vi "SDCP Transfer Mode Command.vi"(4 "error in (no error)":errorcluster, 5 "FTOR":bool, 6 "BTR":bool, 7 "SFT":bool) -> (0 "error out":errorcluster)   [LabVIEW 2020]
uses:
  Typedefs/SDCP - Serial Port Control - Commands.ctl
  <vilib>/Instr/_visa.llb/VISA Flush IO Buffer Mask.ctl
panel:
  out "Number of tries":i32
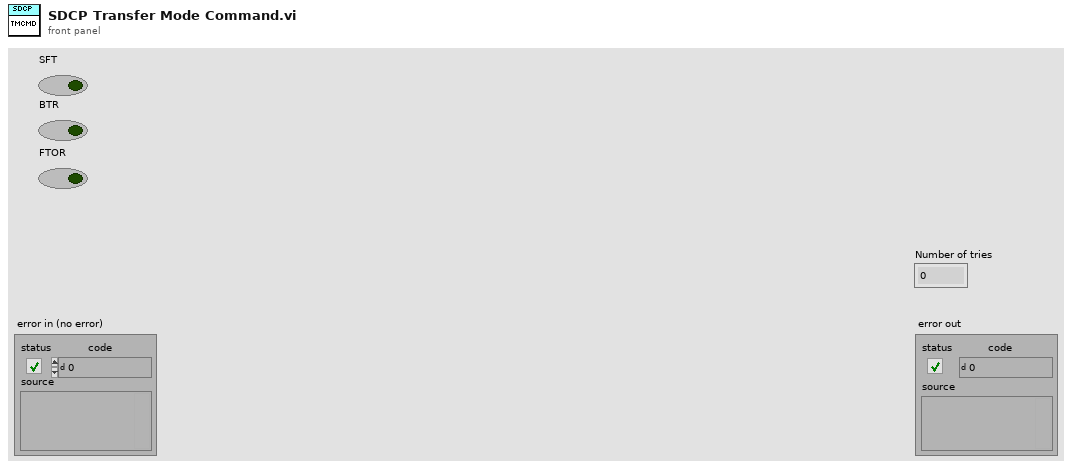
[diagram p1: front panel]
types:
  T1 = typedef "VISA Flush IO Buffer Mask.ctl" = u16
  T2 = typedef "SDCP - Serial Port Control - Commands.ctl" = enum16{"Open", "Read", "Write", "Get instance", "Close"}
  T3 = typedef "SDCP TMC Param.ctl" = cluster{"TMS_REQ":bool, "TMS_ACK":bool, "TMC_REQ":bool, "TMC_ACK":bool, "BTR_ENSTAT":bool, "FTOR_ENSTAT":bool, "SFT_ENSTAT":bool, "BTR_ENREQ":bool, "FTOR_ENREQ":bool, "SFT_ENREQ":bool, "MTR_ENREQ":bool, "MTR_ENACK":bool}
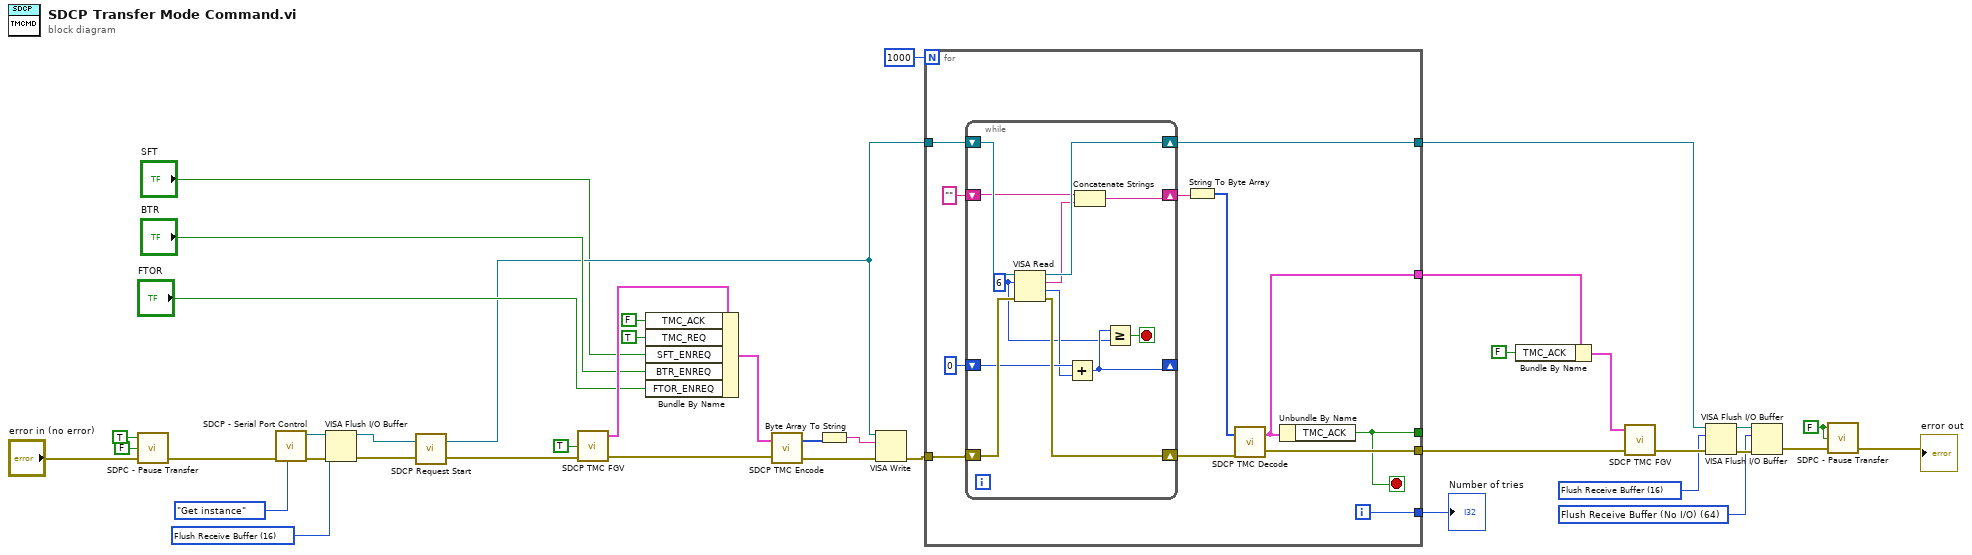
[diagram p0: block diagram]
diagram:
  w2 = FALSE ("Pause transfer")
  w13 = T1 64 items=["Flush Receive Buffer"=16, "Write Transmit Buffer to Device"=32, "Flush Receive Buffer (No I/O)"=64, "Flush Transmit Buffer"=128] ("Mask")
  w16 = T1 16 items=["Flush Receive Buffer"=16, "Write Transmit Buffer to Device"=32, "Flush Receive Buffer (No I/O)"=64, "Flush Transmit Buffer"=128] ("Mask")
  w19 = T1 16 items=["Flush Receive Buffer"=16, "Write Transmit Buffer to Device"=32, "Flush Receive Buffer (No I/O)"=64, "Flush Transmit Buffer"=128] ("Mask")
  n1 = call "SDPC - Pause Transfer.vi"("error in (no error)"="error in (no error)", "RD/nWR"=FALSE, "Pause transfer"=TRUE) -> ("error out"=w10:errorcluster)  [unwired: 1 in, 1 out]
  n2 = call "SDCP - Serial Port Control.vi"("Command"=SDCP_-_Serial_Port_Control_-_Commands."Get instance", "error in (no error)"=w10) -> ("error out"=w21:errorcluster, "VISA out"=w20:refnum<visa-resource-name>)  [unwired: 6 in, 2 out]
  n3 = VISA Flush I/O Buffer(VISA resource name=w20, mask (16)=w19, error in (no error)=w21) -> (VISA resource name out=w6:refnum<visa-resource-name>, error out=w7:errorcluster)
  n4 = call "SDCP Request Start.vi"("error in (no error)"=w7, "COM Port"=w6) -> ("error out"=w4:errorcluster, "COM Port Out"=w5:refnum<visa-resource-name>)
  n5 = call "SDCP TMC FGV.vi"("error in (no error)"=w4, "RD/nWR"=TRUE) -> ("error out"=w33:errorcluster, "TMC out"=w38:T3)  [unwired: 2 in]
  n6 = Bundle By Name(cluster=w38, "TMC_ACK"=FALSE, "TMC_REQ"=TRUE, "SFT_ENREQ"="SFT", "BTR_ENREQ"="BTR", "FTOR_ENREQ"="FTOR") -> (w32:T3)
  n7 = call "SDCP TMC Encode.vi"("error in (no error)"=w33, "SDCP TMC Param"=w32) -> ("error out"=w30:errorcluster, "Encoded frame"=w31:u8[])
  n8 = Byte Array To String(unsigned byte array=w31) -> (string=w29:string)
  n9 = VISA Write(VISA resource name=w5, write buffer=w29, error in (no error)=w30) -> (error out=w28:errorcluster)  [unwired: 2 out]
  n10 = for {
    N: 1000 -> [_]
    tunnel: w28 -> [w52]
    tunnel: w5 -> [w51]
    tunnel: [w45] -> w26
    tunnel: [w44] -> w27
    tunnel: [w42] -> _
    tunnel: [w43] -> w22
    tunnel: [w41] -> w17
    i -> [w43]
    stop <- w42 stop-if-true
    n11 = while {
      shift-right: [w63] -> w48
      shift-left: w52 -> [w64]
      shift-right: [w55] -> _
      shift-left: u32 0 -> [w60]
      shift-right: [w61] -> w41
      shift-left: w51 -> [w62]
      shift-right: [w56] -> w47
      shift-left: "" -> [w58]
      stop <- w54 stop-if-true
      w53 = u32 6 ("byte count")
      n12 = VISA Read(VISA resource name=w62, byte count=w53, error in (no error)=w64) -> (VISA resource name out=w61:refnum<visa-resource-name>, read buffer=w57:string, return count=w59:u32, error out=w63:errorcluster)
      n13 = Add(x=w60, y=w59) -> (x+y=w55:u32)
      n14 = Concatenate Strings(w58, w57) -> (w56:string)
      n15 = Greater Or Equal?(x=w55, y=w53) -> (x >= y?=w54:bool)
    }
    n16 = String To Byte Array(string=w47) -> (unsigned byte array=w46:u8[])
    n17 = call "SDCP TMC Decode.vi"("error in (no error)"=w48, "Frame"=w46) -> ("error out"=w44:errorcluster, "SDCP TMC out"=w45:T3)
    n18 = Unbundle By Name(w45) -> ("TMC_ACK"=w42:bool)
  }
  "Number of tries" <- w22
  n19 = Bundle By Name(cluster=w26, "TMC_ACK"=FALSE) -> (w24:T3)
  n20 = call "SDCP TMC FGV.vi"("error in (no error)"=w27, "TMC in"=w24) -> ("error out"=w18:errorcluster)  [unwired: 2 in, 1 out]
  n21 = VISA Flush I/O Buffer(VISA resource name=w17, mask (16)=w16, error in (no error)=w18) -> (VISA resource name out=w14:refnum<visa-resource-name>, error out=w15:errorcluster)
  n22 = VISA Flush I/O Buffer(VISA resource name=w14, mask (16)=w13, error in (no error)=w15) -> (error out=w9:errorcluster)  [unwired: 1 out]
  n23 = call "SDPC - Pause Transfer.vi"("error in (no error)"=w9, "RD/nWR"=w2, "Pause transfer"=w2) -> ("error out"=→"error out":errorcluster)  [unwired: 1 in, 1 out]
